vi "Broadcast Status.vi"(8 "error in":errorcluster, 10 "Reply Payload":T1) -> (0 "error out":errorcluster)   [LabVIEW 2020, in "Manipulator.lvlib"]
doc: "Get the Status of the Manipulator.\n_____\nCreated using DQMH Event Scripter 6.0.0.122."
uses:
  Manipulator.lvlib
  Get Status (Reply Payload)--cluster.ctl
  Manipulator-CLIDriver/Manipulator Status.ctl
  Manipulator-CLIDriver/Manipulator CLI Driver.lvlib
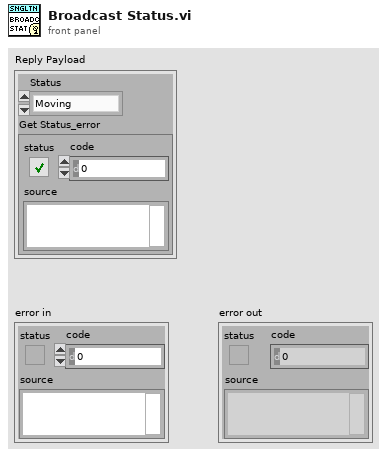
[diagram p1: front panel]
types:
  T1 = typedef "Manipulator.lvlib/Get Status (Reply Payload)--cluster.ctl" = cluster{"Status":T2, "Get Status_error":errorcluster}
  T2 = typedef "Manipulator CLI Driver.lvlib/Manipulator Status.ctl" = enum16{"Moving", "Done", "Aborted", "Error", "No Status"}
  T3 = typedef "Manipulator.lvlib/Broadcast Events--cluster.ctl" = cluster{"Module Did Init":refnum<user-event>, "Status Updated":refnum<user-event>, "Error Reported":refnum<user-event>, "Module Did Stop":refnum<user-event>, "Update Module Execution Status":refnum<user-event>, "Broadcast Num Axes":refnum<user-event>, "Broadcast Position and Speed":refnum<user-event>, "Broadcast Status":refnum<user-event>}
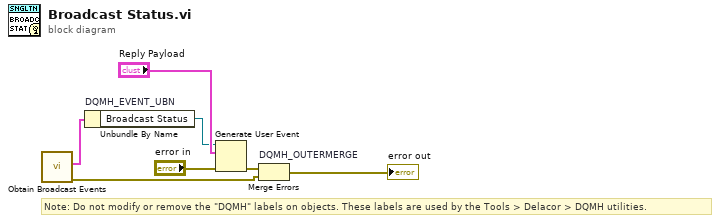
[diagram p0: block diagram]
diagram:
  # "Note: Do not modify or remove the \"DQMH\" labels on objects. These labels are used by the Tools > Delacor > DQMH utilities."
  n1 = call "Obtain Broadcast Events.vi"() -> ("error out"=w2:errorcluster, "Manipulator Broadcast Events"=w1:T3)  [unwired: 10 in]
  n2 = Unbundle By Name "DQMH_EVENT_UBN"(w1) -> ("Broadcast Status"=w4:refnum<user-event>)
  n3 = Generate User Event(user event=w4, event data cluster="Reply Payload", error in="error in") -> (error out=w3:errorcluster)  [unwired: 1 in, 1 out]
  n4 = Merge Errors "DQMH_OUTERMERGE"(w3, w2) -> (→"error out":errorcluster)
